vi "Rectangle Converter.vi"(10 "Scale Factor":dbl=1.0, 11 "Rect":T2) -> (2 "Rect Out":T1, 3 "Center":cluster{"x":dbl, "y":dbl})   [LabVIEW 2016]
doc: "Converts a rectangle defined by top-left point and height and width to a rectangle defined by top-left and bottom-right points. Will also scale the rectangle by the given factor. (All scaling occurs around the original center point.)"
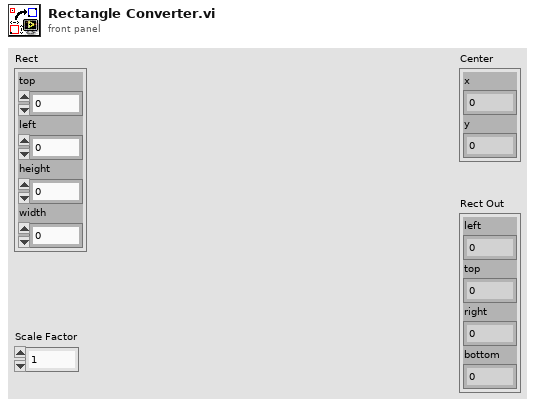
[diagram p1: front panel]
types:
  T1 = cluster{"left":dbl, "top":dbl, "right":dbl, "bottom":dbl}
  T2 = cluster{"top":dbl, "left":dbl, "height":dbl, "width":dbl}
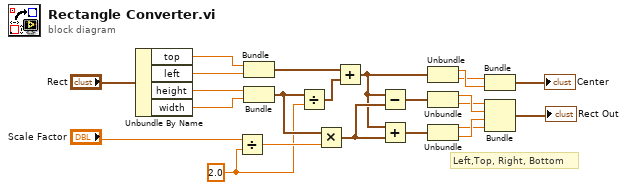
[diagram p0: block diagram]
diagram:
  w1 = 2.0 ("y")
  # "Left,Top, Right, Bottom"
  n1 = Unbundle By Name("Rect") -> ("top"=w22:dbl, "left"=w21:dbl, "height"=w20:dbl, "width"=w19:dbl)
  n2 = Divide(x="Scale Factor", y=w1) -> (x/y=w7:dbl)
  n3 = Bundle("top"=w22, "left"=w21) -> (w9:cluster{"top":dbl, "left":dbl})  [unwired: 1 in]
  n4 = Bundle("height"=w20, "width"=w19) -> (w10:cluster{"height":dbl, "width":dbl})  [unwired: 1 in]
  n5 = Divide(x=w10, y=w1) -> (x/y=w6:cluster{"height":dbl, "width":dbl})
  n6 = Multiply(x=w10, y=w7) -> (x*y=w18:cluster{"height":dbl, "width":dbl})
  n7 = Add(x=w9, y=w6) -> (x+y=w5:cluster{dbl, dbl})
  n8 = Subtract(x=w5, y=w18) -> (x-y=w17:cluster{dbl, dbl})
  n9 = Add(x=w5, y=w18) -> (x+y=w16:cluster{dbl, dbl})
  n10 = Unbundle(w5) -> (w4:dbl, w3:dbl)
  n11 = Unbundle(w17) -> (w15:dbl, w14:dbl)
  n12 = Unbundle(w16) -> (w12:dbl, w13:dbl)
  n13 = Bundle(w3, w4) -> (→"Center":cluster{dbl, dbl})  [unwired: 1 in]
  n14 = Bundle(w14, w15, w13, w12) -> (→"Rect Out":cluster{dbl, dbl, dbl, dbl})  [unwired: 1 in]
